vi "ZAlign_SetWindowSize.vi"(8 "error in (no error)":errorcluster, 10 "rect":T1, 11 "VI in":refnum<vi>) -> (0 "error out":errorcluster, 3 "reference out":refnum<vi>)   [LabVIEW 2014, in "ZAlign.lvlib"]
doc: "ZAlign.lvlib:ZAlign_SetWindowSize.vi\n----------------------------------------------\nCalculate and set Windowsize\n\nInputs:\n---------------------\n- error in (no error) : Cluster; \n- rect : Cluster; \n- VI in : Refnum; \n\nOutputs:\n---------------------\n- error out : Cluster; \n- reference out : Refnum; \n\n----------------------------------------------\n16/03/2015\nZühlke Engineering AG\nCH-8952 Schlieren\nwww.zuehlke.com"
uses:
  ZAlign.lvlib
panel:
  # "Connector Pane"
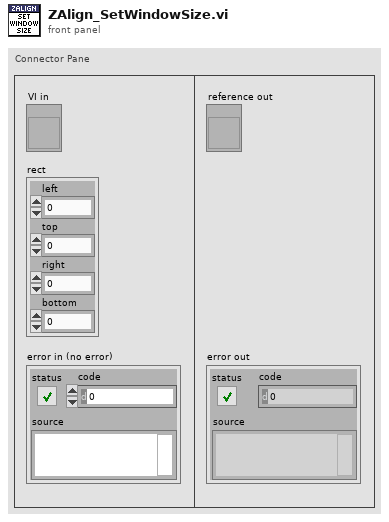
[diagram p1: front panel]
types:
  T1 = cluster{"left":i16, "top":i16, "right":i16, "bottom":i16}
  T2 = typedef "LVRectTypeDef.ctl" = cluster{"Left":i16, "Top":i16, "Right":i16, "Bottom":i16}
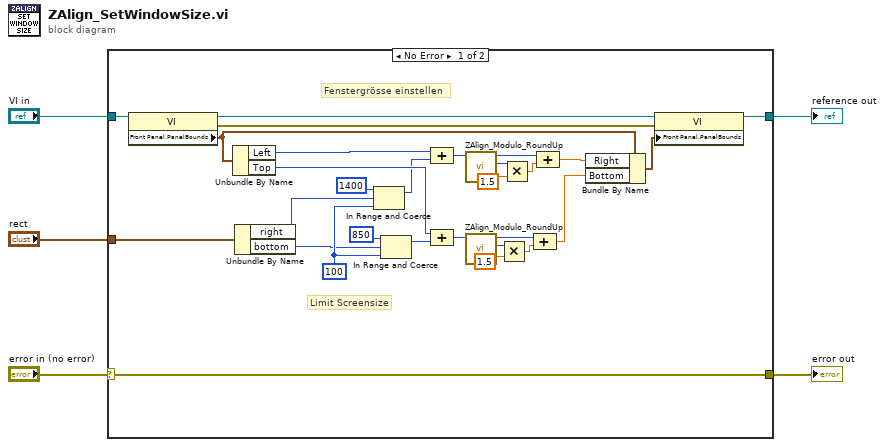
[diagram p0: block diagram]
diagram:
  n1 = case shown="No Error" "error in (no error)" {
    selector: "error in (no error)" -> [w21 w36]
    tunnel: "VI in" -> [w34 w35]
    tunnel: "rect" -> [w26 _]
    tunnel: [w22 w35] -> w3
    tunnel: [w21 w36] -> w1
    frame No Error {
      w16 = 100 ("upper limit")
      # "Limit Screensize"
      # "Fenstergrösse einstellen"
      n2 = property class="VI"(reference=w34) -> (reference out=w23:refnum<vi>, error out=w24:errorcluster, "Front Panel.PanelBounds"=w27:T2)  [unwired: 1 in]
      n3 = Unbundle By Name(w27) -> ("Left"=w28:i16, "Top"=w29:i16)
      n4 = Unbundle By Name(w26) -> ("right"=w13:i16, "bottom"=w15:i16)
      n5 = In Range and Coerce(upper limit=1400, x=w13, lower limit=w16) -> (coerced(x)=w12:i32)  [unwired: 1 out]
      n6 = In Range and Coerce(upper limit=850, x=w15, lower limit=w16) -> (coerced(x)=w14:i32)  [unwired: 1 out]
      n7 = Compound Arithmetic op=ADD(w28, w12) -> (w30:i32)
      n8 = Compound Arithmetic op=ADD(w29, w14) -> (w31:i32)
      n9 = call "ZAlign_Modulo_RoundUp.vi"("Value in"=w30) -> ("Grid_Size"=w11:i32, "Value out"=w32:i32)  [unwired: 9 in]
      n10 = call "ZAlign_Modulo_RoundUp.vi"("Value in"=w31) -> ("Grid_Size"=w7:i32, "Value out"=w33:i32)  [unwired: 9 in]
      n11 = Multiply(x=w7, y=1.5) -> (x*y=w6:dbl)
      n12 = Multiply(x=w11, y=1.5) -> (x*y=w9:dbl)
      n13 = Compound Arithmetic op=ADD(w33, w6) -> (w19:dbl)
      n14 = Compound Arithmetic op=ADD(w32, w9) -> (w20:dbl)
      n15 = Bundle By Name(cluster=w27, "Right"=w20, "Bottom"=w19) -> (w25:T2)
      n16 = property class="VI"(reference=w23, error in=w24, "Front Panel.PanelBounds"=w25) -> (reference out=w22:refnum<vi>)  [unwired: 1 out]
    }
    frame Error {
    }
  }
  "reference out" <- w3
  "error out" <- w1
